vi "Check Callback.vi"(5 "Config VI Ref":refnum<vi>, 6 "Create Callback?":bool, 7 "Parent VI Ref":refnum<vi>, 9 "Error Message Ref":refnum<vi>, 10 "Warning Icon Ref":refnum<vi>, 11 "Callback Path":string) -> (3 "Valid Callback?":bool)   [LabVIEW 2021]
uses:
  <vilib>/myRIO/Common/Instrument Driver Framework/myRIO v1.0/IRQ/typedefs/Callback VI Ref.ctl
  <vilib>/myRIO/Express VI/IRQ/Message Globals.vi
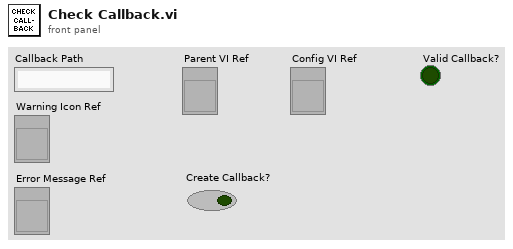
[diagram p1: front panel]
types:
  T1 = typedef "Callback VI Ref.ctl" = refnum<vi>
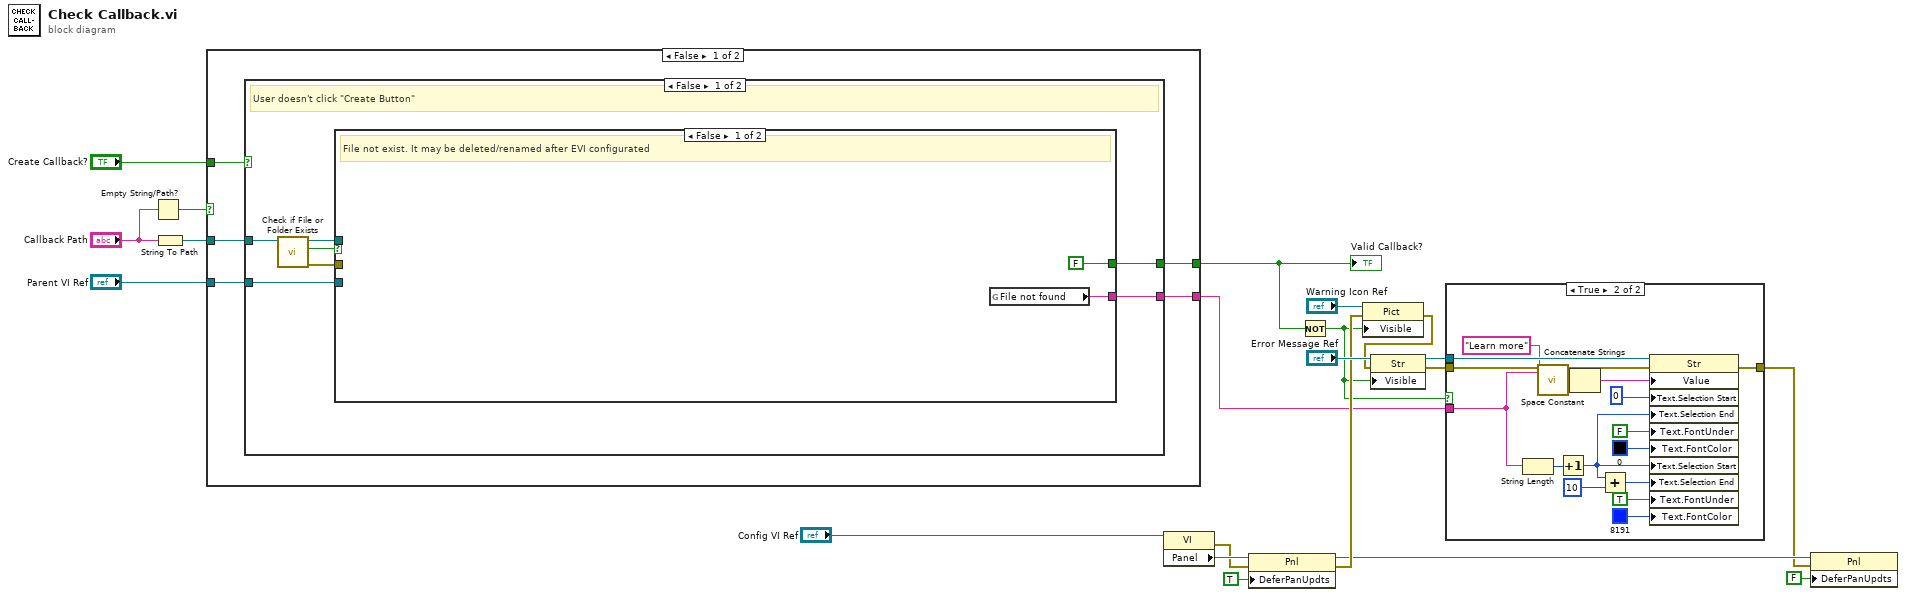
[diagram p0: block diagram]
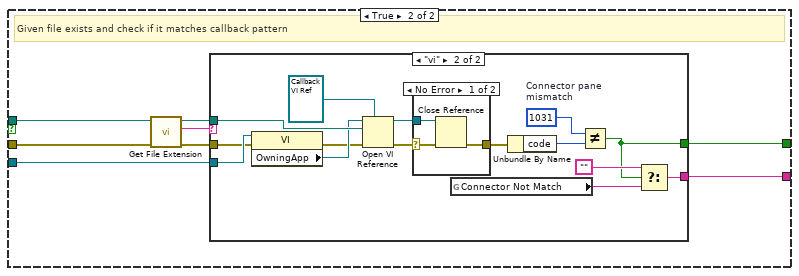
[diagram p3: hidden frame]
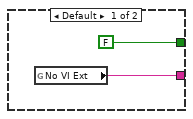
[diagram p4: hidden frame]
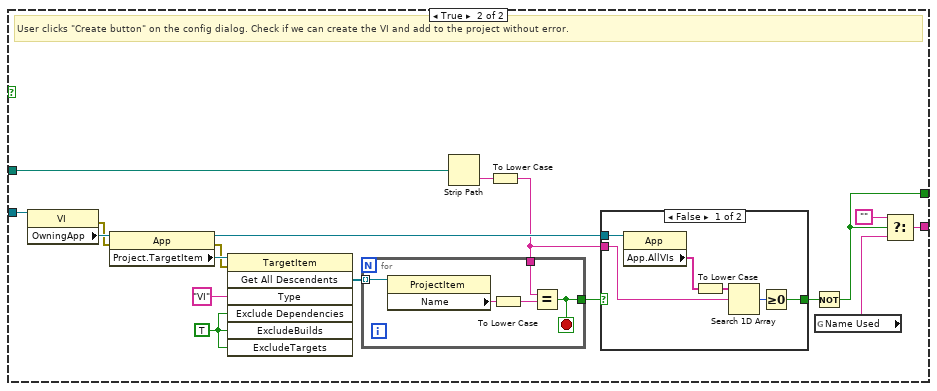
[diagram p6: hidden frame]
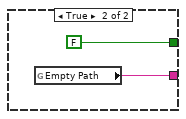
[diagram p8: hidden frame]
diagram:
  n1 = Empty String/Path?(string/path="Callback Path") -> (empty?=w2:bool)
  n2 = String To Path(string="Callback Path") -> (path=w4:path)
  n3 = case shown="False" w2 {
    tunnel: [w26 FALSE] -> w20
    tunnel: [w25 w96] -> w10
    tunnel: "Parent VI Ref" -> [w24 _]
    tunnel: w4 -> [w22 _]
    tunnel: "Create Callback?" -> [w23 _]
    frame False {
      n4 = case shown="False" w23 {
        tunnel: w22 -> [w29 w82]
        tunnel: [w33 w65] -> w26
        tunnel: [w32 w81] -> w25
        tunnel: w24 -> [w31 w80]
        frame False {
          # "User doesn't click \"Create Button\""
          n5 = call <vilib>:"Check if File or Folder Exists.vi"("path"=w29) -> ("error out"=w28:errorcluster, "file or folder exists?"=w27:bool, "dup path"=w30:path)  [unwired: 8 in]
          n6 = case shown="False" w27 {
            tunnel: [FALSE w43] -> w33
            tunnel: [w34 w42] -> w32
            tunnel: w31 -> [_ w41]
            tunnel: w30 -> [_ w40]
            tunnel: w28 -> [_ w36]
            frame False {
              # "File not exist. It may be deleted/renamed after EVI configurated"
              n7 = global read "Message Globals.vi" "File not found"() -> (w34:string)
            }
            frame True {
              # "Given file exists and check if it matches callback pattern"
              n8 = call <vilib>:"Get File Extension.vi"("error in (no error)"=w36, "file"=w40) -> ("error out"=w38:errorcluster, "lowercase file extension"=w37:string, "dup file"=w39:path)  [unwired: 5 in, 2 out]
              n9 = case shown="\"vi\"" w37 {
                tunnel: w39 -> [_ w56]
                tunnel: w38 -> [_ w50]
                tunnel: [FALSE w46] -> w43
                tunnel: [w44 w53] -> w42
                tunnel: w41 -> [_ w52]
                frame Default {
                  n10 = global read "Message Globals.vi" "No VI Ext"() -> (w44:string)
                }
                frame "vi" {
                  w47 = 1031  # Connector pane  mismatch
                  n11 = property class="VI"(reference=w52, error in=w50) -> (error out=w49:errorcluster, "OwningApp"=w51:refnum<vi>)  [unwired: 1 out]
                  n12 = Open VI Reference(type specifier VI Refnum (for type only)=T1 refnum ("Callback VI"), application reference (local)=w51, vi path=w56, error in (no error)=w49) -> (vi reference=w58:T1, error out=w59:errorcluster)  [unwired: 2 in]
                  n13 = case shown="No Error" w59 {
                    selector: w59 -> [w63 w64]
                    tunnel: w58 -> [w61 _]
                    tunnel: [w62 w64] -> w57
                    frame No Error {
                      n14 = Close Reference(reference=w61, error in (no error)=w63) -> (error out=w62:errorcluster)
                    }
                    frame Error {
                    }
                  }
                  n15 = global read "Message Globals.vi" "Connector Not Match"() -> (w54:string)
                  n16 = Unbundle By Name(w57) -> ("code"=w48:i32)
                  n17 = Not Equal?(x=w47, y=w48) -> (x != y?=w46:bool)
                  n18 = Select(t="", s=w46, f=w54) -> (s? t:f=w53:string)
                }
              }
            }
          }
        }
        frame True {
          w76 = TRUE ("ExcludeDependencies")
          # "User clicks \"Create button\" on the config dialog. Check if we can create the VI and add to the project without error."
          n19 = property class="VI"(reference=w80) -> (error out=w71:errorcluster, "OwningApp"=w79:refnum<vi>)  [unwired: 1 in, 1 out]
          n20 = property class="App"(reference=w79, error in=w71) -> (reference out=w69:refnum<vi>, error out=w72:errorcluster, "Project.TargetItem"=w73:refnum<vi>)
          n21 = invoke class="TargetItem" method="Get All Descendents"(reference=w73, error in=w72, "Type"="VI", "Exclude Dependencies"=w76, "ExcludeBuilds"=w76, "ExcludeTargets"=w76) -> ("All Descendents"=w74:refnum<vi>[])  [unwired: 1 in, 6 out]
          n22 = Strip Path(path=w82) -> (name=w68:string)  [unwired: 1 out]
          n23 = To Lower Case(string=w68) -> (all lower case string=w67:string)
          n24 = for {
            tunnel: w74 -> [w94] mode=indexing
            tunnel: w67 -> [w92]
            tunnel: [w91] -> w70
            stop <- w91 stop-if-true
            n25 = property class="ProjectItem"(reference=w94) -> ("Name"=w93:string)  [unwired: 1 in, 2 out]
            n26 = To Lower Case(string=w93) -> (all lower case string=w90:string)
            n27 = Equal?(x=w92, y=w90) -> (x = y?=w91:bool)
          }
          n28 = case shown="False" w70 {
            selector: w70 -> [_ w89]
            tunnel: w69 -> [w88 _]
            tunnel: w67 -> [w85 _]
            tunnel: [w83 w89] -> w66
            frame False {
              n29 = property class="App"(reference=w88) -> ("App.AllVIs"=w84:string[])  [unwired: 1 in, 2 out]
              n30 = To Lower Case(string=w84) -> (all lower case string=w87:string[])
              n31 = Search 1D Array(1D array=w87, element=w85) -> (index of element=w86:i32)  [unwired: 1 in]
              n32 = Greater Or Equal To 0?(x=w86) -> (x >= 0?=w83:bool)
            }
            frame True {
            }
          }
          n33 = Not(x=w66) -> (.not. x?=w65:bool)
          n34 = global read "Message Globals.vi" "Name Used"() -> (w77:string)
          n35 = Select(t="", s=w65, f=w77) -> (s? t:f=w81:string)
        }
      }
    }
    frame True {
      n36 = global read "Message Globals.vi" "Empty Path"() -> (w96:string)
    }
  }
  "Valid Callback?" <- w20
  n37 = property class="VI"(reference="Config VI Ref") -> (error out=w11:errorcluster, "Panel"=w16:refnum<vi>)  [unwired: 1 in, 1 out]
  n38 = property class="Pnl"(reference=w16, error in=w11, "DeferPanUpdts"=TRUE ("Defer Panel Updates")) -> (reference out=w12:refnum<vi>, error out=w13:errorcluster)
  n39 = Not(x=w20) -> (.not. x?=w5:bool)
  n40 = property class="Pict"(reference="Warning Icon Ref", error in=w13, "Visible"=w5) -> (error out=w7:errorcluster)  [unwired: 1 out]
  n41 = property class="Str"(reference="Error Message Ref", error in=w7, "Visible"=w5) -> (reference out=w9:refnum<vi>, error out=w6:errorcluster)
  n42 = case shown="True" w5 {
    tunnel: w6 -> [w97 w113]
    tunnel: w10 -> [_ w110]
    tunnel: w9 -> [_ w106]
    tunnel: [w97 w105] -> w8
    frame False {
    }
    frame True {
      n43 = String Length(string=w110) -> (length=w103:i32)
      n44 = call <vilib>:"Space Constant.vi"() -> ("String"=w99:string)
      n45 = Increment(x=w103) -> (x+1=w98:i32)
      n46 = Concatenate Strings(w110, w99, "Learn more") -> (w109:string)
      n47 = Add(x=w98, y=10) -> (x+y=w102:i32)
      n48 = property class="Str"(reference=w106, error in=w113, "Value"=w109, "Text.Selection Start"=u32 0 ("Text.Selection:Start"), "Text.Selection End"=w98, "Text.FontUnder"=FALSE ("Text.Font:Underline"), "Text.FontColor"=u32 0 ("Text.Text Colors:Text Color"), "Text.Selection Start"=w98, "Text.Selection End"=w102, "Text.FontUnder"=TRUE ("Text.Font:Underline"), "Text.FontColor"=u32 8191 ("Text.Text Colors:Text Color")) -> (error out=w105:errorcluster)  [unwired: 1 out]
    }
  }
  n49 = property class="Pnl"(reference=w12, error in=w8, "DeferPanUpdts"=FALSE ("Defer Panel Updates")) -> ()  [unwired: 2 out]
